vi "Main.vi"(8 "error in (no error)":errorcluster, 11 "Data Server Thread in":refnum<class "Data Server Thread.lvclass">) -> (0 "error out":errorcluster, 3 "Data Server Thread out":refnum<class "Data Server Thread.lvclass">)   [LabVIEW 2017, in "DSF Core.lvlib" / "Data Server Thread.lvclass"]
uses:
  Data Server Thread.lvclass
  C:/Git/DSF/Core/Classes/Thread/Plugin/Plugin Thread.lvclass
  C:/Git/DSF/Core/Classes/Thread/Thread.lvclass
  Plugin/Plugin Thread.lvclass/Plugin Thread.ctl
  Interfaces/Interface/Interface.lvclass/Interface.ctl
  Interfaces/Plugin/Response Data.ctl
  Interfaces/Plugin/Response.ctl
  Interfaces/Plugin/Response Parameters.ctl
  Interfaces/Plugin/Wait For.vi
  Interfaces/Plugin/Wait For Plugin Command.vi
  Transceiver/Get Interface.vi
  Interfaces/Interface/Wait For Command.vi
  Interfaces/Interface/Read RT FIFO.vi
  Interfaces/Plugin/Plugin Interface.lvclass
  C:/Git/DSF/Core/Classes/Interfaces/Interface/Interface.lvclass
  Interfaces/Plugin/Class Name.vi
  VIs/VI Name.vi
  Interfaces/Interface/Errors.vi
  Interfaces/Dispatcher/Command Timeout.vi
  Plugin/Plugin Thread.lvclass
  Thread.lvclass
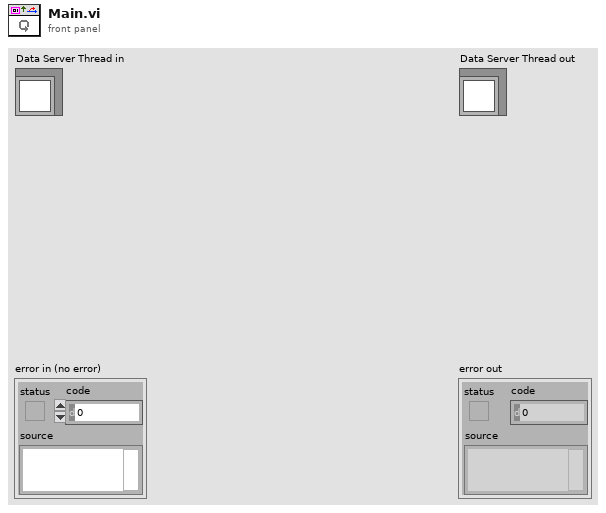
[diagram p1: front panel]
types:
  T1 = typedef "DSF Core.lvlib/Plugin Interface.lvclass/Response Data.ctl" = cluster{"Response":T2, "Parameters":T3}
  T2 = typedef "DSF Core.lvlib/Plugin Interface.lvclass/Response.ctl" = enum8{"General Ack", "Shutting Down"}
  T3 = typedef "DSF Core.lvlib/Plugin Interface.lvclass/Response Parameters.ctl" = cluster{"arg1":u64, "arg2":u64}
  T4 = typedef "DSF Core.lvlib/Plugin Interface.lvclass/Command Data.ctl" = cluster{"Command":T5, "Parameters":T6}
  T5 = typedef "DSF Core.lvlib/Plugin Interface.lvclass/Command.ctl" = enum8{"Start", "Set Inline Buffer", "Rx", "Tx", "Shutdown"}
  T6 = typedef "DSF Core.lvlib/Plugin Interface.lvclass/Command Parameters.ctl" = cluster{"arg1":u64, "arg2":u64}
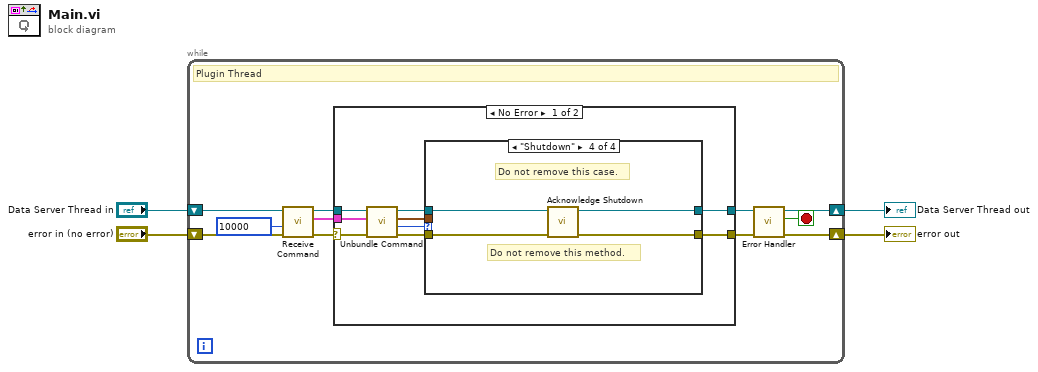
[diagram p0: block diagram]
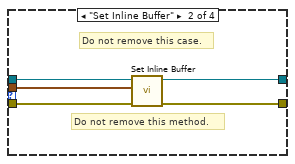
[diagram p3: hidden frame]
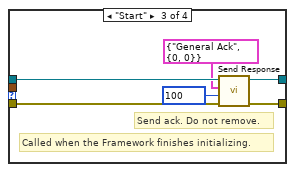
[diagram p4: hidden frame]
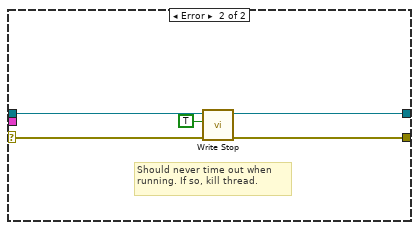
[diagram p5: hidden frame]
diagram:
  n1 = while {
    shift-right: [w10] -> w4
    shift-left: "error in (no error)" -> [w15]
    shift-right: [w11] -> w3
    shift-left: "Data Server Thread in" -> [w14]
    stop <- w9 stop-if-true
    # "Plugin Thread"
    n2 = call "Receive Command.vi"("error in (no error)"=w15, "timeout in ms (0)"=10000 ("timeout in ms"), "Plugin Thread in"=w14) -> ("error out"=w5:errorcluster, "command"=w6:T4, "Plugin Thread out"=w7:refnum<class "Data Server Thread.lvclass">)  [unwired: 6 in]
    n3 = case shown="No Error" w5 {
      selector: w5 -> [w16 w45]
      tunnel: w7 -> [w22 w46]
      tunnel: [w24 w42] -> w13
      tunnel: w6 -> [w21 _]
      tunnel: [w23 w44] -> w12
      frame No Error {
        n4 = call "Unbundle Command.vi"("error in (no error)"=w16, "command"=w21, "Plugin Thread in"=w22) -> ("error out"=w19:errorcluster, "command"=w20:T5, "command parameters"=w17:T6, "Plugin Thread out"=w18:refnum<class "Data Server Thread.lvclass">)  [unwired: 5 in]
        n5 = case shown="\"Shutdown\"" w20 {
          tunnel: w18 -> [w26 w31 w36 w41]
          tunnel: [w26 w30 w35 w39] -> w24
          tunnel: w19 -> [w25 w27 w32 w40]
          tunnel: w17 -> [_ w28 _ _]
          tunnel: [w25 w29 w34 w38] -> w23
          frame Default {
          }
          frame "Set Inline Buffer" {
            # "Do not remove this method."
            # "Do not remove this case."
            n6 = call "Set Inline Buffer.vi"("error in (no error)"=w27, "command parameters"=w28, "Plugin Thread in"=w31) -> ("error out"=w29:errorcluster, "Plugin Thread out"=w30:refnum<class "Data Server Thread.lvclass">)  [unwired: 7 in]
          }
          frame "Start" {
            # "Send ack. Do not remove."
            # "Called when the Framework finishes initializing."
            n7 = call "Send Response.vi"("error in (no error)"=w32, "timeout in ms (0)"=100, "response"=T1 {"Response"=enum."General Ack", "Parameters"={"arg1"=0, "arg2"=0}}, "Plugin Thread in"=w36) -> ("error out"=w34:errorcluster, "Plugin Thread out"=w35:refnum<class "Data Server Thread.lvclass">)  [unwired: 6 in]
          }
          frame "Shutdown" {
            # "Do not remove this method."
            # "Do not remove this case."
            n8 = call "Acknowledge Shutdown.vi"("error in (no error)"=w40, "Plugin Thread in"=w41) -> ("error out"=w38:errorcluster, "Plugin Thread out"=w39:refnum<class "Data Server Thread.lvclass">)  [unwired: 8 in]
          }
        }
      }
      frame Error {
        # "Should never time out when running. If so, kill thread."
        n9 = call "Write Stop.vi"("error in (no error)"=w45, "stop"=TRUE, "Thread in"=w46) -> ("error out"=w44:errorcluster, "Thread out"=w42:refnum<class "Data Server Thread.lvclass">)  [unwired: 7 in]
      }
    }
    n10 = call "Error Handler.vi"("error in (no error)"=w12, "Plugin Thread in"=w13) -> ("error out"=w10:errorcluster, "stop"=w9:bool, "Plugin Thread out"=w11:refnum<class "Data Server Thread.lvclass">)  [unwired: 7 in]
  }
  "error out" <- w4
  "Data Server Thread out" <- w3
